vi "WriteToPannelAddressSpace.vi"(6 "Scratch Output Values":i32[](array[numeric]), 8 "error in (no error)":errorcluster, 9 "Digital Write Values":bool[](array[boolean]), 10 "Analog Write Values":i32[](array[numeric]), 11 "comms cluster in":T1) -> (0 "error out":errorcluster, 3 "comms cluster out":T1)   [LabVIEW 2025]
doc: "Writes all program outputs to corresponding\nMB discrete coils and registers.\n\nINPUTS:\n 1. comms cluster of:\n a) station reg start address\n b)16-bit modulo of local user IP\n c) MB comms line \n 2. Analog output array -- 8x1 array of type int\n to write to output reg associated with panel\n output AO-0 -> AO-7\n 3. Digital output array -- 8x1 array of type bool\n to write to output coils associated with panel\n output DO-0 -> DO-7 \n 4. comms error line\n 5. Scratch output values -- MB server\n registers associated with interapplication\n comms. -- e.g.: transaction of information\n between MATLAB and this VI.\n\nOUTPUTS:\n 1. repackaged comms cluster of:\n a) station reg start address\n b)16-bit modulo of local user IP\n c) MB comms line \n 2. comms error line"
uses:
  <vilib>/Modbus/master/Modbus Master.lvclass
panel:
  # "Write all pannel registers and contacts\n\nWrites all program outputs to corresponding\nMB discrete coils and registers.\n\nINPUTS:\n  1. comms cluster of:\n      a) station reg start address\n      b)16-bit modulo of local user IP\n      c) MB comms line \n   2. Analog output array -- 8x1 array of type int\n       to write to output reg associated with panel\n       output AO-0 -> AO-7\n   3. Digital output array -- 8x1 array of type bool\n       to write to output coils associated with panel\n       output DO-0 -> DO-7 \n   4. comms error line\n   5. Scratch output values -- MB server\n       registers associated with interapplication\n       comms. -- e.g.: transaction of information\n       between MATLAB and this VI.\n\nOUTPUTS:\n   1. repackaged comms cluster of:\n      a) station reg start address\n      b)16-bit modulo of local user IP\n      c) MB comms line \n   2. comms error line"
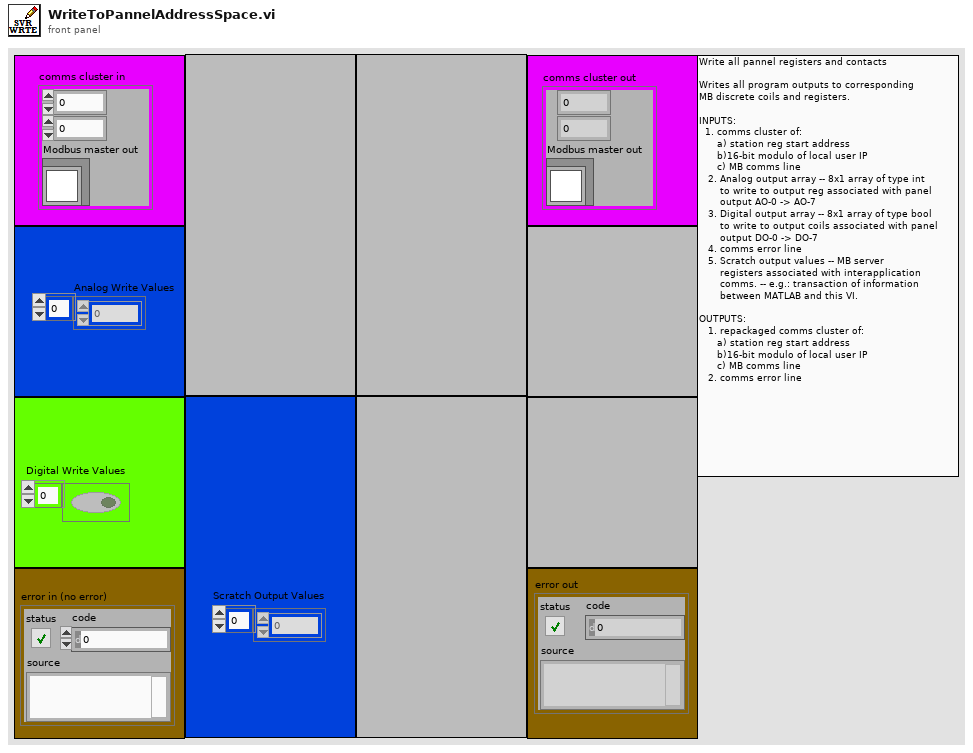
[diagram p1: front panel]
types:
  T1 = cluster{u16, u32, "Modbus master out":refnum<class "Modbus Master.lvclass">}
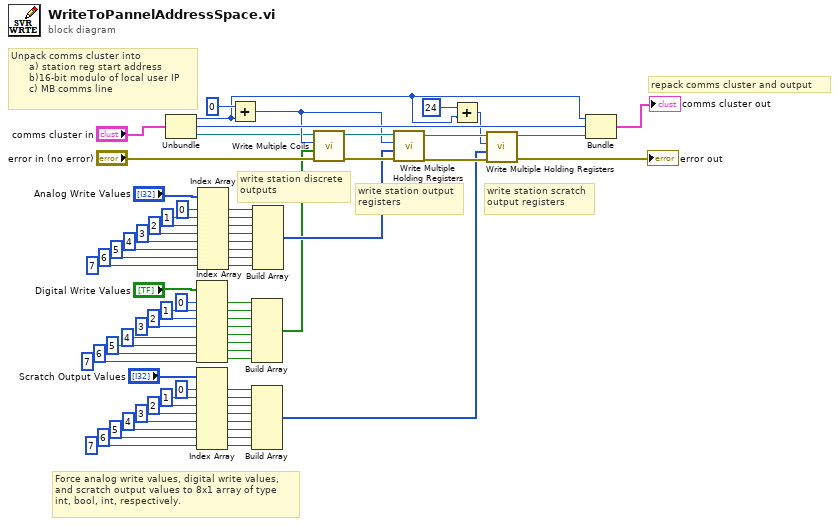
[diagram p0: block diagram]
diagram:
  # "write station discrete\noutputs"
  # "write station scratch\noutput registers"
  # "write station output\nregisters"
  # "repack comms cluster and output"
  # "Unpack comms cluster into\n      a) station reg start address\n      b)16-bit modulo of local user IP\n      c) MB comms line"
  # "Force analog write values, digital write values, \nand scratch output values to 8x1 array of type\nint, bool, int, respectively."
  n1 = Unbundle("comms cluster in") -> (w10:u16, w67:u32, "Modbus master out"=w46:refnum<class "Modbus Master.lvclass">)
  n2 = Index Array(array="Digital Write Values", index #1=0 ("index"), index #2=1 ("index"), index #3=2 ("index"), index #4=3 ("index"), index #5=4 ("index"), index #6=5 ("index"), index #7=6 ("index"), index #8=7 ("index")) -> (element #1=w40:bool, element #2=w41:bool, element #3=w42:bool, element #4=w43:bool, element #5=w4:bool, element #6=w3:bool, element #7=w2:bool, element #8=w1:bool)
  n3 = Index Array(array="Scratch Output Values", index #1=0 ("index"), index #2=1 ("index"), index #3=2 ("index"), index #4=3 ("index"), index #5=4 ("index"), index #6=5 ("index"), index #7=6 ("index"), index #8=7 ("index")) -> (element #1=w18:i32, element #2=w17:i32, element #3=w16:i32, element #4=w15:i32, element #5=w27:i32, element #6=w28:i32, element #7=w29:i32, element #8=w30:i32)
  n4 = Index Array(array="Analog Write Values", index #1=0 ("index"), index #2=1 ("index"), index #3=2 ("index"), index #4=3 ("index"), index #5=4 ("index"), index #6=5 ("index"), index #7=6 ("index"), index #8=7 ("index")) -> (element #1=w50:i32, element #2=w49:i32, element #3=w48:i32, element #4=w47:i32, element #5=w59:i32, element #6=w60:i32, element #7=w61:i32, element #8=w62:i32)
  n5 = Add(x=u16 0, y=w10) -> (x+y=w63:u16)
  n6 = Build Array(w40, w41, w42, w43, w4, w3, w2, w1) -> (w44:bool[])
  n7 = Build Array(w18, w17, w16, w15, w27, w28, w29, w30) -> (w8:i32[])
  n8 = Build Array(w50, w49, w48, w47, w59, w60, w61, w62) -> (w65:i32[])
  n9 = call-dynamic "Write Multiple Coils.vi"("error in (no error)"="error in (no error)", "coil values"=w44, "starting address"=w63, "Modbus master in"=w46) -> ("error out"=w66:errorcluster, "Modbus master out"=w64:refnum<class "Modbus Master.lvclass">)  [unwired: 6 in]
  n10 = call-dynamic "Write Multiple Holding Registers.vi"("error in (no error)"=w66, "holding register values"=w65, "starting address"=w63, "Modbus master in"=w64) -> ("error out"=w12:errorcluster, "Modbus master out"=w13:refnum<class "Modbus Master.lvclass">)  [unwired: 6 in]
  n11 = Add(x=u16 24, y=w10) -> (x+y=w9:u16)
  n12 = call-dynamic "Write Multiple Holding Registers.vi"("error in (no error)"=w12, "holding register values"=w8, "starting address"=w9, "Modbus master in"=w13) -> ("error out"=→"error out":errorcluster, "Modbus master out"=w7:refnum<class "Modbus Master.lvclass">)  [unwired: 6 in]
  n13 = Bundle(w10, w67, "Modbus master out"=w7) -> (→"comms cluster out":T1)  [unwired: 1 in]
